vi "setUp.vi"(8 "error in (no error)":errorcluster, 11 "reference in":refnum<class "Action Update Set Point.lvclass">) -> (0 "error out":errorcluster, 3 "reference out":refnum<class "Action Update Set Point.lvclass">)   [LabVIEW 2018, in "Action Update Set Point.lvclass"]
doc: "setUp runs prior to the test method during test execution. Use this method to initialize any object data required by your tests."
uses:
  Action Update Set Point.lvclass
  E:/Program Files (x86)/National Instruments/Circuit Design Suite 14.1/LabVIEW 2018/vi.lib/addons/_JKI Toolkits/VI Tester/TestCase.llb/TestCase.lvclass
  Action Update Set Point.lvclass/Action Update Set Point.ctl
  <vilib>/addons/_JKI Toolkits/VI Tester/TestCase.llb/TestCase.lvclass
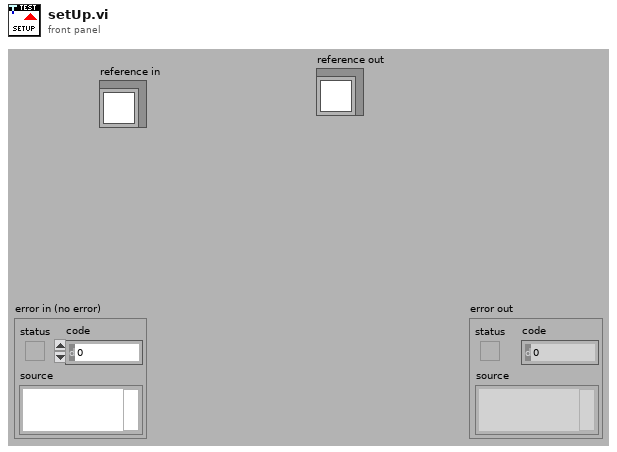
[diagram p1: front panel]
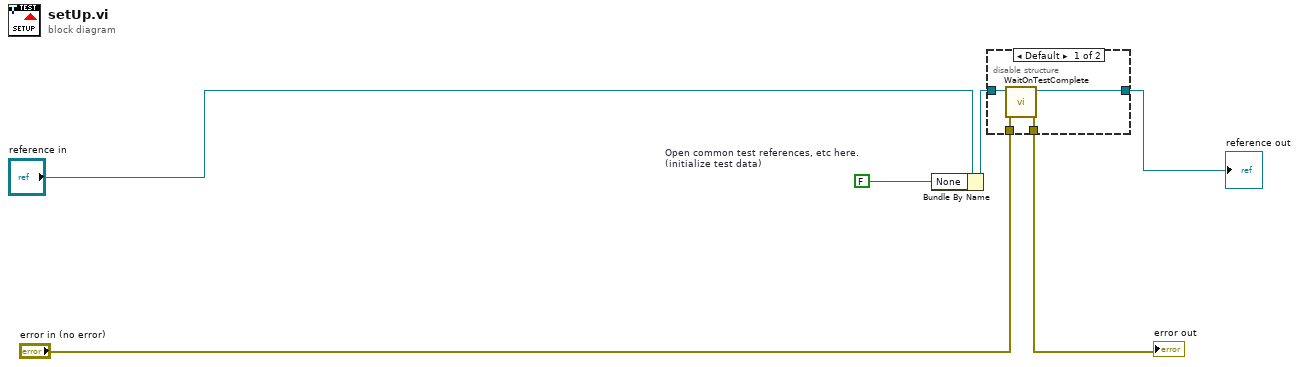
[diagram p0: block diagram]
diagram:
  w3 = FALSE  # Open common test references, etc here. (initialize test data)
  n1 = Bundle By Name(cluster="reference in", "None"=w3) -> (w4:refnum<class "Action Update Set Point.lvclass">)
  n2 = disable-structure shown="Default" {
    disable-tunnel: "error in (no error)" -> [w10 w11]
    disable-tunnel: [w9 w11] -> w5
    disable-tunnel: [w8 w12] -> w1
    disable-tunnel: w4 -> [w7 w12]
    frame condition #0 (active) {
      n3 = call <vilib>:"WaitOnTestComplete.vi"("error in (no error)"=w10, "TestCase in"=w7) -> ("error out"=w9:errorcluster, "TestCase out"=w8:refnum<class "Action Update Set Point.lvclass">)  [unwired: 8 in]
    }
    frame condition #1 {
    }
  }
  "error out" <- w5
  "reference out" <- w1
